vi "HRM-AQN-myDAQ_read.vi"(8 "error in (no error)":errorcluster, 11 "AQN cluster in":T1) -> (0 "error out":errorcluster, 2 "data":waveform(dbl), 3 "AQN cluster out":T1)   [LabVIEW 2020]
uses:
  HRM-AQN-input_clust.ctl
  <vilib>/DAQmx/read.llb/DAQmx Read (Analog Wfm 1Chan NSamp).vi
  <vilib>/DAQmx/miscellaneous.llb/DAQmx Fill In Error Info.vi
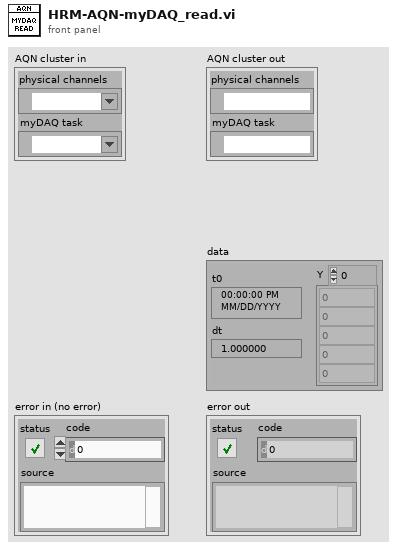
[diagram p1: front panel]
types:
  T1 = typedef "HRM-AQN-input_clust.ctl" = cluster{"physical channels":tag, "myDAQ task":refnum<k21>}
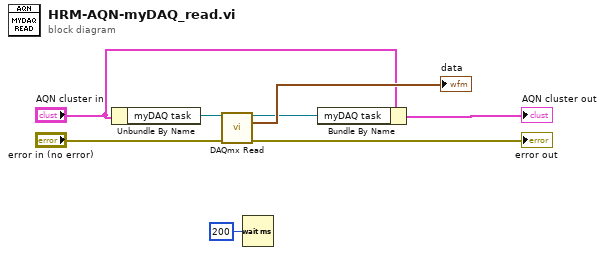
[diagram p0: block diagram]
diagram:
  n1 = Unbundle By Name("AQN cluster in") -> ("myDAQ task"=w4:refnum<k21>)
  n2 = call-poly <vilib>:"DAQmx Read.vi"("task/channels in"=w4, "error in"="error in (no error)") -> ("task out"=w5:refnum<k21>, "data"=→"data":waveform(dbl), "error out"=→"error out":errorcluster)  [unwired: 11 in]
  n3 = Wait (ms)(milliseconds to wait=u32 200) -> ()  [unwired: 1 out]
  n4 = Bundle By Name(cluster="AQN cluster in", "myDAQ task"=w5) -> (→"AQN cluster out":T1)
